vi "gyro -- async sweeper.vi"(8 "win":T3={"cen (Hz)"=45005.0594236074, "win (Hz)"=127.23590686512762, "left (Hz)"=44941.44147017484, "right (Hz)"=45068.67737703997}, 10 "sweeper talkback":refnum<user-event>, 11 "sweeper talkto":refnum<user-event>) -> ()   [LabVIEW 2018]
uses:
  gyro -- async sweeper parameters.ctl
  freq scan type.ctl
  pll sweeper talkto message type.ctl
  pll sweeper talkback message type.ctl
  show-win- control.ctl
  publisher action.ctl
  data source action.ctl
  array - generate range.vi
  array -- sort 2D array -- Complex.vi/05c44075-957c-bc42-b6fa-2799d0bc0485.vi
  <vilib>/Array/Sort 2D Array - Pop Stack.vi
  <vilib>/Array/Sort 2D Array - Push Stack.vi
panel:
  out "Numeric":i32
  in  "Tab Control":enum32{"Page 1", "Page 2"}(tab)
  in  "sweeper parameters":T1={"delay-circle(msec)"=0, "N"=250, "scan type"=enum."linear", "gamma factor"=2378.60310421286, "history length"=0}
  out "stop!":bool
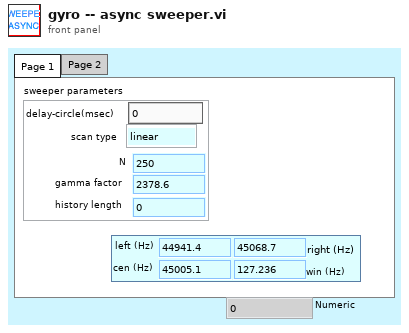
[diagram p1: front panel]
types:
  T1 = typedef "gyro -- async sweeper parameters.ctl" = cluster{"delay-circle(msec)":i64, "N":i64, "scan type":T2, "gamma factor":dbl, "history length":i64}
  T2 = typedef "freq scan type.ctl" = enum16{"linear", "arctan"}
  T3 = typedef "show-win- control.ctl" = cluster{"cen (Hz)":dbl, "win (Hz)":dbl, "left (Hz)":dbl, "right (Hz)":dbl}
  T4 = typedef "data source action.ctl" = enum16{"set", "get", "init", "set-and-get", "init source"}
  T5 = typedef "publisher action.ctl" = enum16{"set", "get", "init", "check"}
  T6 = typedef "pll sweeper talkback message type.ctl" = cluster{"message":enum16{"new"}}
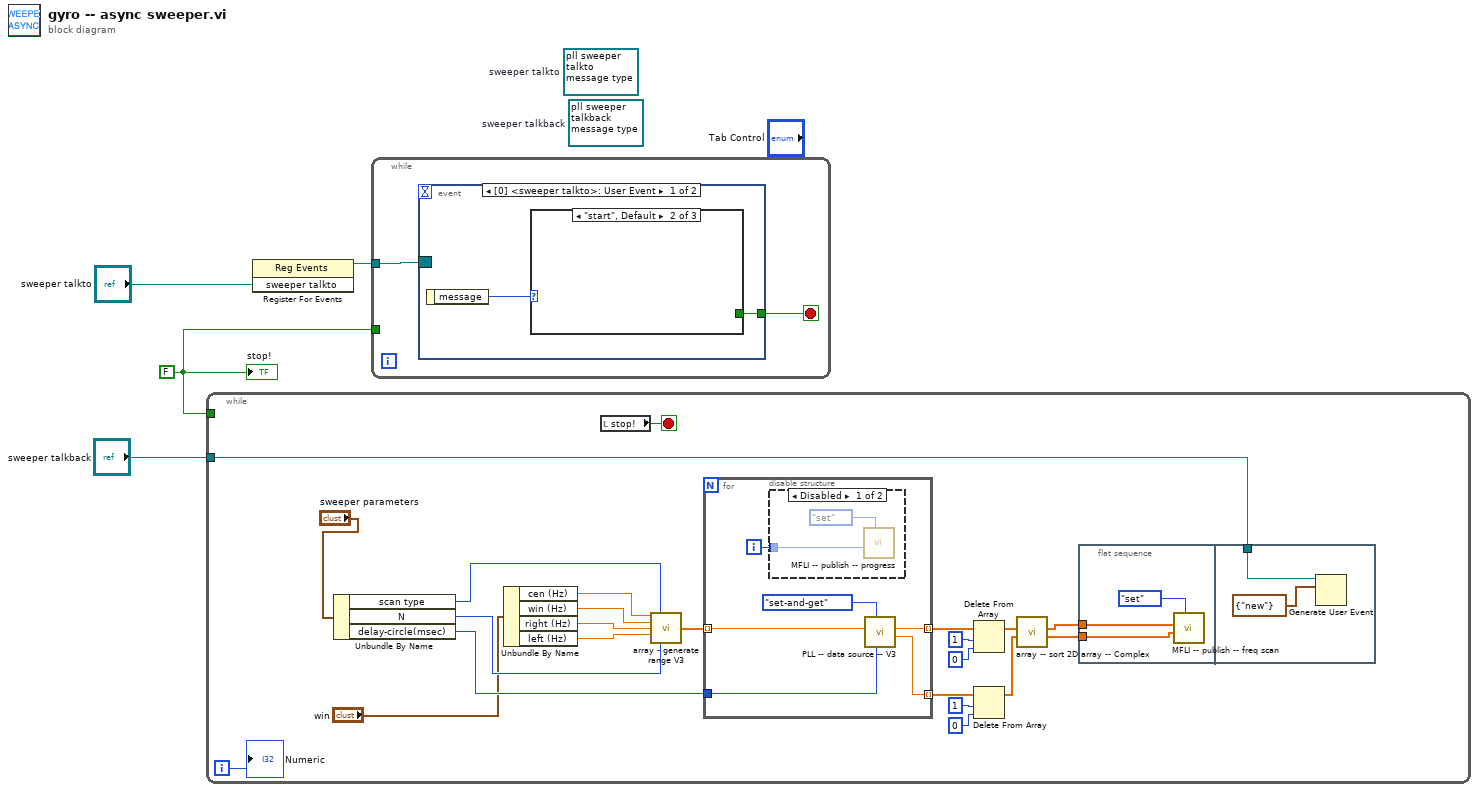
[diagram p0: block diagram]
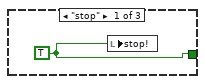
[diagram p2: hidden frame]
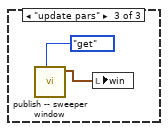
[diagram p3: hidden frame]
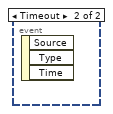
[diagram p4: hidden frame]
diagram:
  (unwired) refnum<user-event> refnum  # sweeper talkback
  (unwired) refnum<user-event> refnum  # sweeper talkto
  w3 = FALSE ("stop!")
  n1 = while {
    tunnel: w3 -> [_]
    tunnel: "sweeper talkback" -> [w15]
    i -> [w5]
    stop <- w16 stop-if-true
    n2 = Unbundle By Name("sweeper parameters") -> ("scan type"=w14:T2, "N"=w7:i64, "delay-circle(msec)"=w8:i64)
    n3 = Unbundle By Name("win") -> ("cen (Hz)"=w12:dbl, "win (Hz)"=w11:dbl, "right (Hz)"=w10:dbl, "left (Hz)"=w9:dbl)
    n4 = local read "stop!"() -> (w16:bool)
    n5 = call "array - generate range V3.vi"("center"=w12, "scan type"=w14, "window"=w11, "freq max"=w10, "freq min"=w9, "N"=w7) -> ("Array"=w13:dbl[])  [unwired: 8 in, 1 out]
    n6 = for {
      tunnel: w13 -> [w28] mode=indexing
      tunnel: w8 -> [w30]
      tunnel: [w33] -> w23 mode=indexing
      tunnel: [w32] -> w22 mode=indexing
      i -> [w31]
      n7 = disable-structure shown="Disabled" {
        disable-tunnel: w31 -> [w34 _]
        frame Disabled {
          n8 = call "MFLI -- publish -- progress.vi"("publisher action"=publisher_action."set", "num"=w34) -> ()  [unwired: 9 in, 1 out]
        }
        frame Enabled {
        }
      }
      n9 = call "PLL -- data source -- V3.vi"("set-get delay (msec)"=w30, "data source action"=data_source_action."set-and-get", "Freq in (Hz)"=w28) -> ("z out (V)"=w33:cdb, "Freq out (Hz)"=w32:dbl)  [unwired: 6 in, 1 out]
    }
    n10 = Delete From Array(array=w22, length=1, index=0) -> (array with subset deleted=w21:dbl[])  [unwired: 1 out]
    n11 = Delete From Array(array=w23, length=1, index=0) -> (array with subset deleted=w20:cdb[])  [unwired: 1 out]
    n12 = call "array -- sort 2D array -- Complex.vi"("z In"=w20, "freq IN"=w21) -> ("z out"=w18:cdb[], "freq out"=w19:dbl[])  [unwired: 8 in]
    n13 = flat-sequence {
      tunnel: w18 -> [w37]
      tunnel: w19 -> [w36]
      tunnel: w15 -> [w40]
      frame #0 {
        n14 = call "MFLI -- publish -- freq scan.vi"("publisher action"=publisher_action."set", "Voltage IN (V)"=w37, "Freq IN (Hz)"=w36) -> ()  [unwired: 7 in, 2 out]
      }
      frame #1 {
        n15 = Generate User Event(user event=w40, event data cluster=T6 {"message"=enum."new"} ("event data")) -> ()  [unwired: 2 in, 2 out]
      }
    }
    "Numeric" <- w5
  }
  n16 = register-events("sweeper talkto") -> (reference out=w4:refnum<event-registration>)  [unwired: 2 in, 1 out]
  n17 = while {
    tunnel: w4 -> [w42]
    tunnel: w3 -> [_]
    stop <- w41 stop-if-true
    n18 = event shown="[0] <sweeper talkto>: User Event" {
      selector: w42 -> [_ _]
      dyn-events: _ -> [_ _]
      timeout: _ -> [_ _]
      tunnel: [w44 _] -> w41
      event User Event {
        n19 = event-data() -> ("message"=w43:enum16{"stop", "start", "update pars"})  [unwired: 1 in]
        n20 = case shown="\"start\", Default" w43 {
          tunnel: [w45 _ _] -> w44
          frame "stop" {
            w45 = TRUE ("stop!")
            n21 = local write "stop!"(w45) -> ()
          }
          frame "start", Default {
          }
          frame "update pars" {
            n22 = call "publish -- sweeper window.vi"("publisher action"=publisher_action."get") -> ("win OUT"=w46:T3)  [unwired: 10 in]
            n23 = local write "win"(w46) -> ()
          }
        }
      }
      event Timeout {
        n24 = event-data() -> ()  [unwired: 1 in, 3 out]
      }
    }
  }
  "stop!" <- w3
